vi "Write Column Information.vi"(8 "error in (no error)":errorcluster, 10 "Column Information":T1, 11 "Column in":refnum<class "Column.lvclass">) -> (0 "error out":errorcluster, 3 "Column out":refnum<class "Column.lvclass">)   [LabVIEW 2020]
uses:
  Column.lvclass
  C:/Users/User/Desktop/Raman Program/Database OOP/source/Database OOP/Basic Columns/Column Class/Column.lvclass
  C:/Users/User/Desktop/Raman Program/Database OOP/source/Database OOP/Column Interface/Column Interface Class/Column Interface.lvclass
  <vilib>/addons/database/Auxilliary.llb/DB Tools DataTypes.ctl
  <vilib>/addons/database/NI_Database_API.lvlib
  Column Interface/Column Information.ctl
  Basic Columns.lvlib
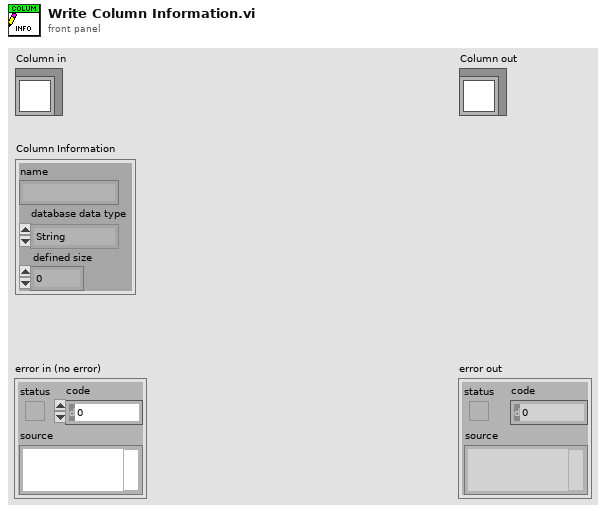
[diagram p1: front panel]
types:
  T1 = typedef "Basic Columns.lvlib/Column Information.ctl" = cluster{"name":string, "database data type":T2, "defined size":i32}
  T2 = typedef "NI_Database_API.lvlib/DB Tools DataTypes.ctl" = enum16{"String", "Long (I32)", "Single (SGL)", "Double (DBL)", "Date/Time", "Binary"}
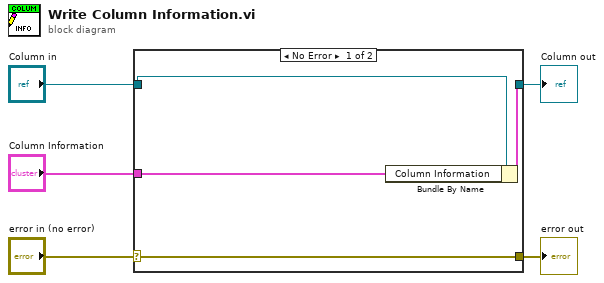
[diagram p0: block diagram]
diagram:
  n1 = case shown="No Error" "error in (no error)" {
    selector: "error in (no error)" -> [w9 w10]
    tunnel: [w9 w10] -> w4
    tunnel: [w7 w11] -> w2
    tunnel: "Column in" -> [w8 w11]
    tunnel: "Column Information" -> [w6 _]
    frame No Error {
      n2 = Bundle By Name(cluster=w8, "Column Information"=w6) -> (w7:cluster{})
    }
    frame Error {
    }
  }
  "error out" <- w4
  "Column out" <- w2
